vi "Do.vi"(8 "error in (no error)":errorcluster, 10 "Actor in":refnum<class "Actor.lvclass">, 11 "New Command Processor Status Msg":refnum<class "New Command Processor Status Msg.lvclass">) -> (0 "error out":errorcluster, 2 "Actor out":refnum<class "Actor.lvclass">)   [LabVIEW 2013, in "System.lvlib" / "New Command Processor Status Msg.lvclass"]
doc: "This VI delivers the message to the actor by calling the appropriate method(s) on the actor."
uses:
  New Command Processor Status Msg.lvclass
  <vilib>/ActorFramework/Actor/Actor.lvclass
  System/System.lvclass
  New Command Processor Status Msg.lvclass/New Command Processor Status Msg.ctl
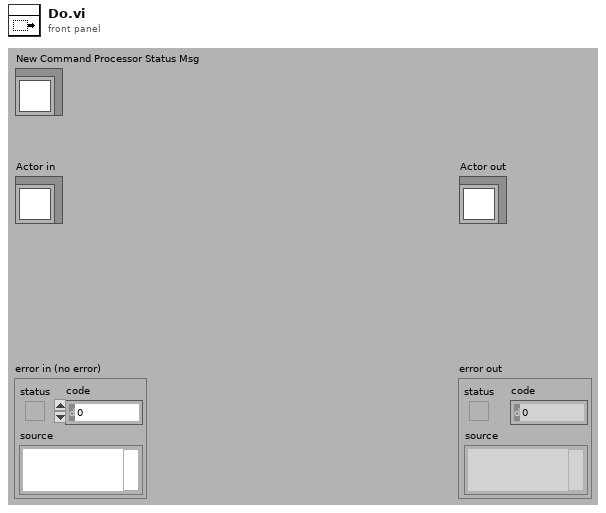
[diagram p1: front panel]
types:
  T1 = typedef "Command Processor.lvlib/Command Processor.lvclass/Command Processor Status.ctl" = cluster{"State Entry time":timestamp, "State Status":T2, "Command Processor Current State":string, "Command Status":T4}
  T2 = typedef "Current Previous State Status.ctl" = cluster{"Current State Status":T3, "Previous State Status":T3}
  T3 = typedef "State Status.ctl" = cluster{"State Name":string, "State Entry Time":timestamp, "State Exit Time":timestamp}
  T4 = typedef "Command Processor.lvlib/Command.lvlib/Command.lvclass/Command Status.ctl" = cluster{"Command Name":string, "Current State Status":T5, "Command Start Time":timestamp, "Command End Time":timestamp, "Previous State Status":T5}
  T5 = typedef "Command Processor.lvlib/Command.lvlib/Command.lvclass/State Status.ctl" = cluster{"State Name":string, "State Entry Time":timestamp, "State Exit Time":timestamp}
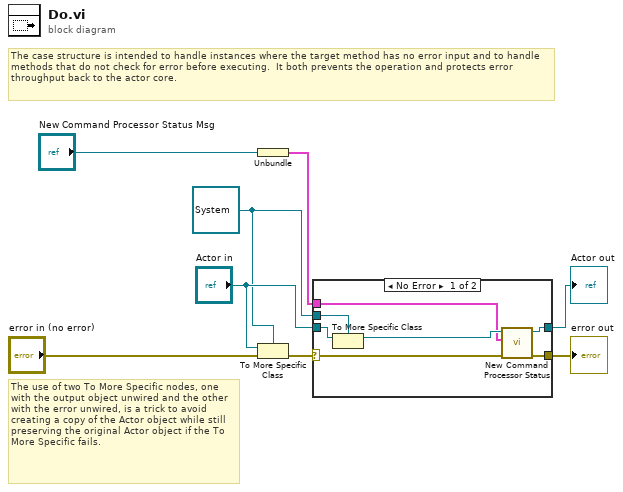
[diagram p0: block diagram]
diagram:
  w2 = refnum<class "System.lvclass"> refnum ("Actor in")
  # "The use of two To More Specific nodes, one with the output object unwired and the other with the error unwired, is a trick to avoid creating a copy of the Actor object while still preserving the original Actor object if the To More Specific fails."
  # "The case structure is intended to handle instances where the target method has no error input and to handle methods that do not check for error before executing.  It both prevents the operation and protects error throughput back to the actor core."
  n1 = Unbundle("New Command Processor Status Msg") -> (w1:T1)
  n2 = To More Specific Class(target class=w2, reference="Actor in", error in="error in (no error)") -> (error out=w6:errorcluster)  [unwired: 1 out]
  n3 = case shown="No Error" w6 {
    selector: w6 -> [w13 w17]
    tunnel: [w15 w17] -> w5
    tunnel: [w14 w16] -> w4
    tunnel: "Actor in" -> [w12 w16]
    tunnel: w2 -> [w11 _]
    tunnel: w1 -> [w9 _]
    frame No Error {
      n4 = To More Specific Class(target class=w11, reference=w12) -> (specific class reference=w10:refnum<class "System.lvclass">)  [unwired: 1 in, 1 out]
      n5 = call-dynamic "New Command Processor Status.vi"("error in (no error)"=w13, "Command Processor Status"=w9, "System in"=w10) -> ("error out"=w15:errorcluster, "System out"=w14:refnum<class "System.lvclass">)  [unwired: 7 in]
    }
    frame Error {
      # "If type check fails, pass the original object out again."
    }
  }
  "error out" <- w5
  "Actor out" <- w4
